vi "Habid_2-D_Histogram_Max_Average_and_Derivate_Beta.vi"() -> ()   [LabVIEW 2009]
uses:
  <vilib>/Analysis/6fits.llb/Curve Fitting Criteria.ctl
  <vilib>/Utility/file.llb/Write To Spreadsheet File (DBL).vi
  <vilib>/Analysis/3filter.llb/Savitzky-Golay Filter (DBL).vi
  <vilib>/Analysis/3filter.llb/Butterworth Filter (DBL).vi
  <vilib>/Analysis/NI_AALBase.lvlib
  <vilib>/Analysis/NI_AALPro.lvlib
  <vilib>/ptbypt/NI_PtbyPt.lvlib
panel:
  out "derivative M.A. 2":cluster{"Filtered X":dbl[], dbl[]}(graph)
  in  "Save 2-D":bool
  in  "Result File Dir 3":path
  in  "Result File Name 3":string="1D_Histogram.txt"
  out "y-axis":dbl[](array[numeric])
  out "S.D.":dbl format="%0.2f"
  in  "AC Mod Gain":dbl=5.0
  out "x-axis":dbl[](array[numeric])
  in  "Save 1-D":bool
  in  "Result File Dir":path
  in  "Result File Name":string="1D_Histogram.txt"
  in  "Save Derivative?":bool
  in  "Result File Dir 2":path
  in  "Result File Name 2":string="1D_Histogram.txt"
  in  "Ramp Rate":dbl=5.0
  out "Individual 2D Histogram":dbl[][](graph)
  out "Total 2D Histogram":dbl[][](graph)
  out "derivative M.A.":cluster{"Value":dbl, dbl, dbl[]}(graph)
  out "Smooth M.A.":cluster{"Value":dbl, dbl, dbl[]}(graph)
  in  "polynomial order 2":i32=3
  in  "side points 2":i32=9
  out "fit for M.A 2":cluster{"Value":dbl, dbl, dbl[][]}(graph)
  out "slope M.A.":dbl
  out "Real Threshold M.A.":cluster{"Value":dbl, dbl, dbl[]}(graph)
  in  "threshold y 2":dbl=-2.0
  out "Threshold 2":cluster{"Value":dbl, dbl, dbl[]}(graph)
  out "fit for M.A.":cluster{"Value":dbl, dbl, dbl[]}(graph)
  out "1-D Histogram M.A.":cluster{dbl[], dbl[]}[](graph)
  in  "Average Max?":bool
  in  "Threshold?":bool
  in  "Derivative?":bool
  out "fit for Max":cluster{"Value":dbl, dbl, dbl[]}(graph)
  out "S.D. Fit":dbl format="%0.5f"
  out "threshold slope":dbl
  out "fit threshold":cluster{dbl, dbl, ext[][]}(graph)
  out "threshold":cluster{dbl, dbl, ext[]}(graph)
  out "mean":dbl format="%0.5f"
  out "slope":dbl
  out "Fit":cluster{dbl, dbl, ext[][]}(graph)
  out "Gain Multiplier I(t)":cluster{dbl, dbl, "Filtered X":dbl[]}(graph)
  out "After I(t)":cluster{dbl, dbl, "Filtered X":dbl[]}(graph)
  out "Before I(t)":cluster{dbl, "SamplingTime":dbl, "Data":ext[]}(graph)
  in  "start path":path=path "J:/data"
  out "NormAC":dbl[](array[numeric])
  in  "Save Curve?":bool
  out "CurrentFileName":string
  out "SelectedCurves":i32
  out "CurvesInHistogram":bool[](array[boolean])
  out "1-D Histogram":cluster{dbl[], dbl[]}(graph)
  in  "1-D Histogram?":bool
  in  "Continuous?":bool
  in  "Add Histogram?":bool
  in  "Current (V) bins":i32=100
  in  "Current (V) max":dbl=2.0
  in  "Current (V) min":dbl=-3.0
  in  "Distance bins":i32=500
  in  "Distance max":dbl=4.0
  in  "Distance min":dbl
  in  "+/-":bool=TRUE
  out "DcData":dbl[](array[numeric])
  out "Beta":dbl[](array[numeric])
  out "DcDataLog":dbl[](array[numeric])
  out "TotalCurves":i32
  out "CurrentCurve":i32
  in  "Next Curve":bool
  in  "Previous Curve":bool
  out "AC I(t)":T1(graph)
  in  "Piezo Sensitivity (nm/V)":dbl=3.89
  in  "Z-mod Amp (V)":dbl=0.0257
  in  "Gac/Gdc":dbl=1.16618
  in  "low cutoff freq: fl":u32=600
  in  "high cutoff freq: fh":u32=1400
  out "DC I(t)":T2(graph)
  in  "DC cutoff freq":i32=1200
  out "Original I(t)":cluster{dbl, "SamplingTime":dbl, "Data":ext[]}(graph)
  out "DataBuffer":dbl[](array[numeric])
  out "Sampling Freq":dbl
  out "Sampling Time":dbl
  out "TimeLine":dbl[](array[numeric])
  in  "stop":bool
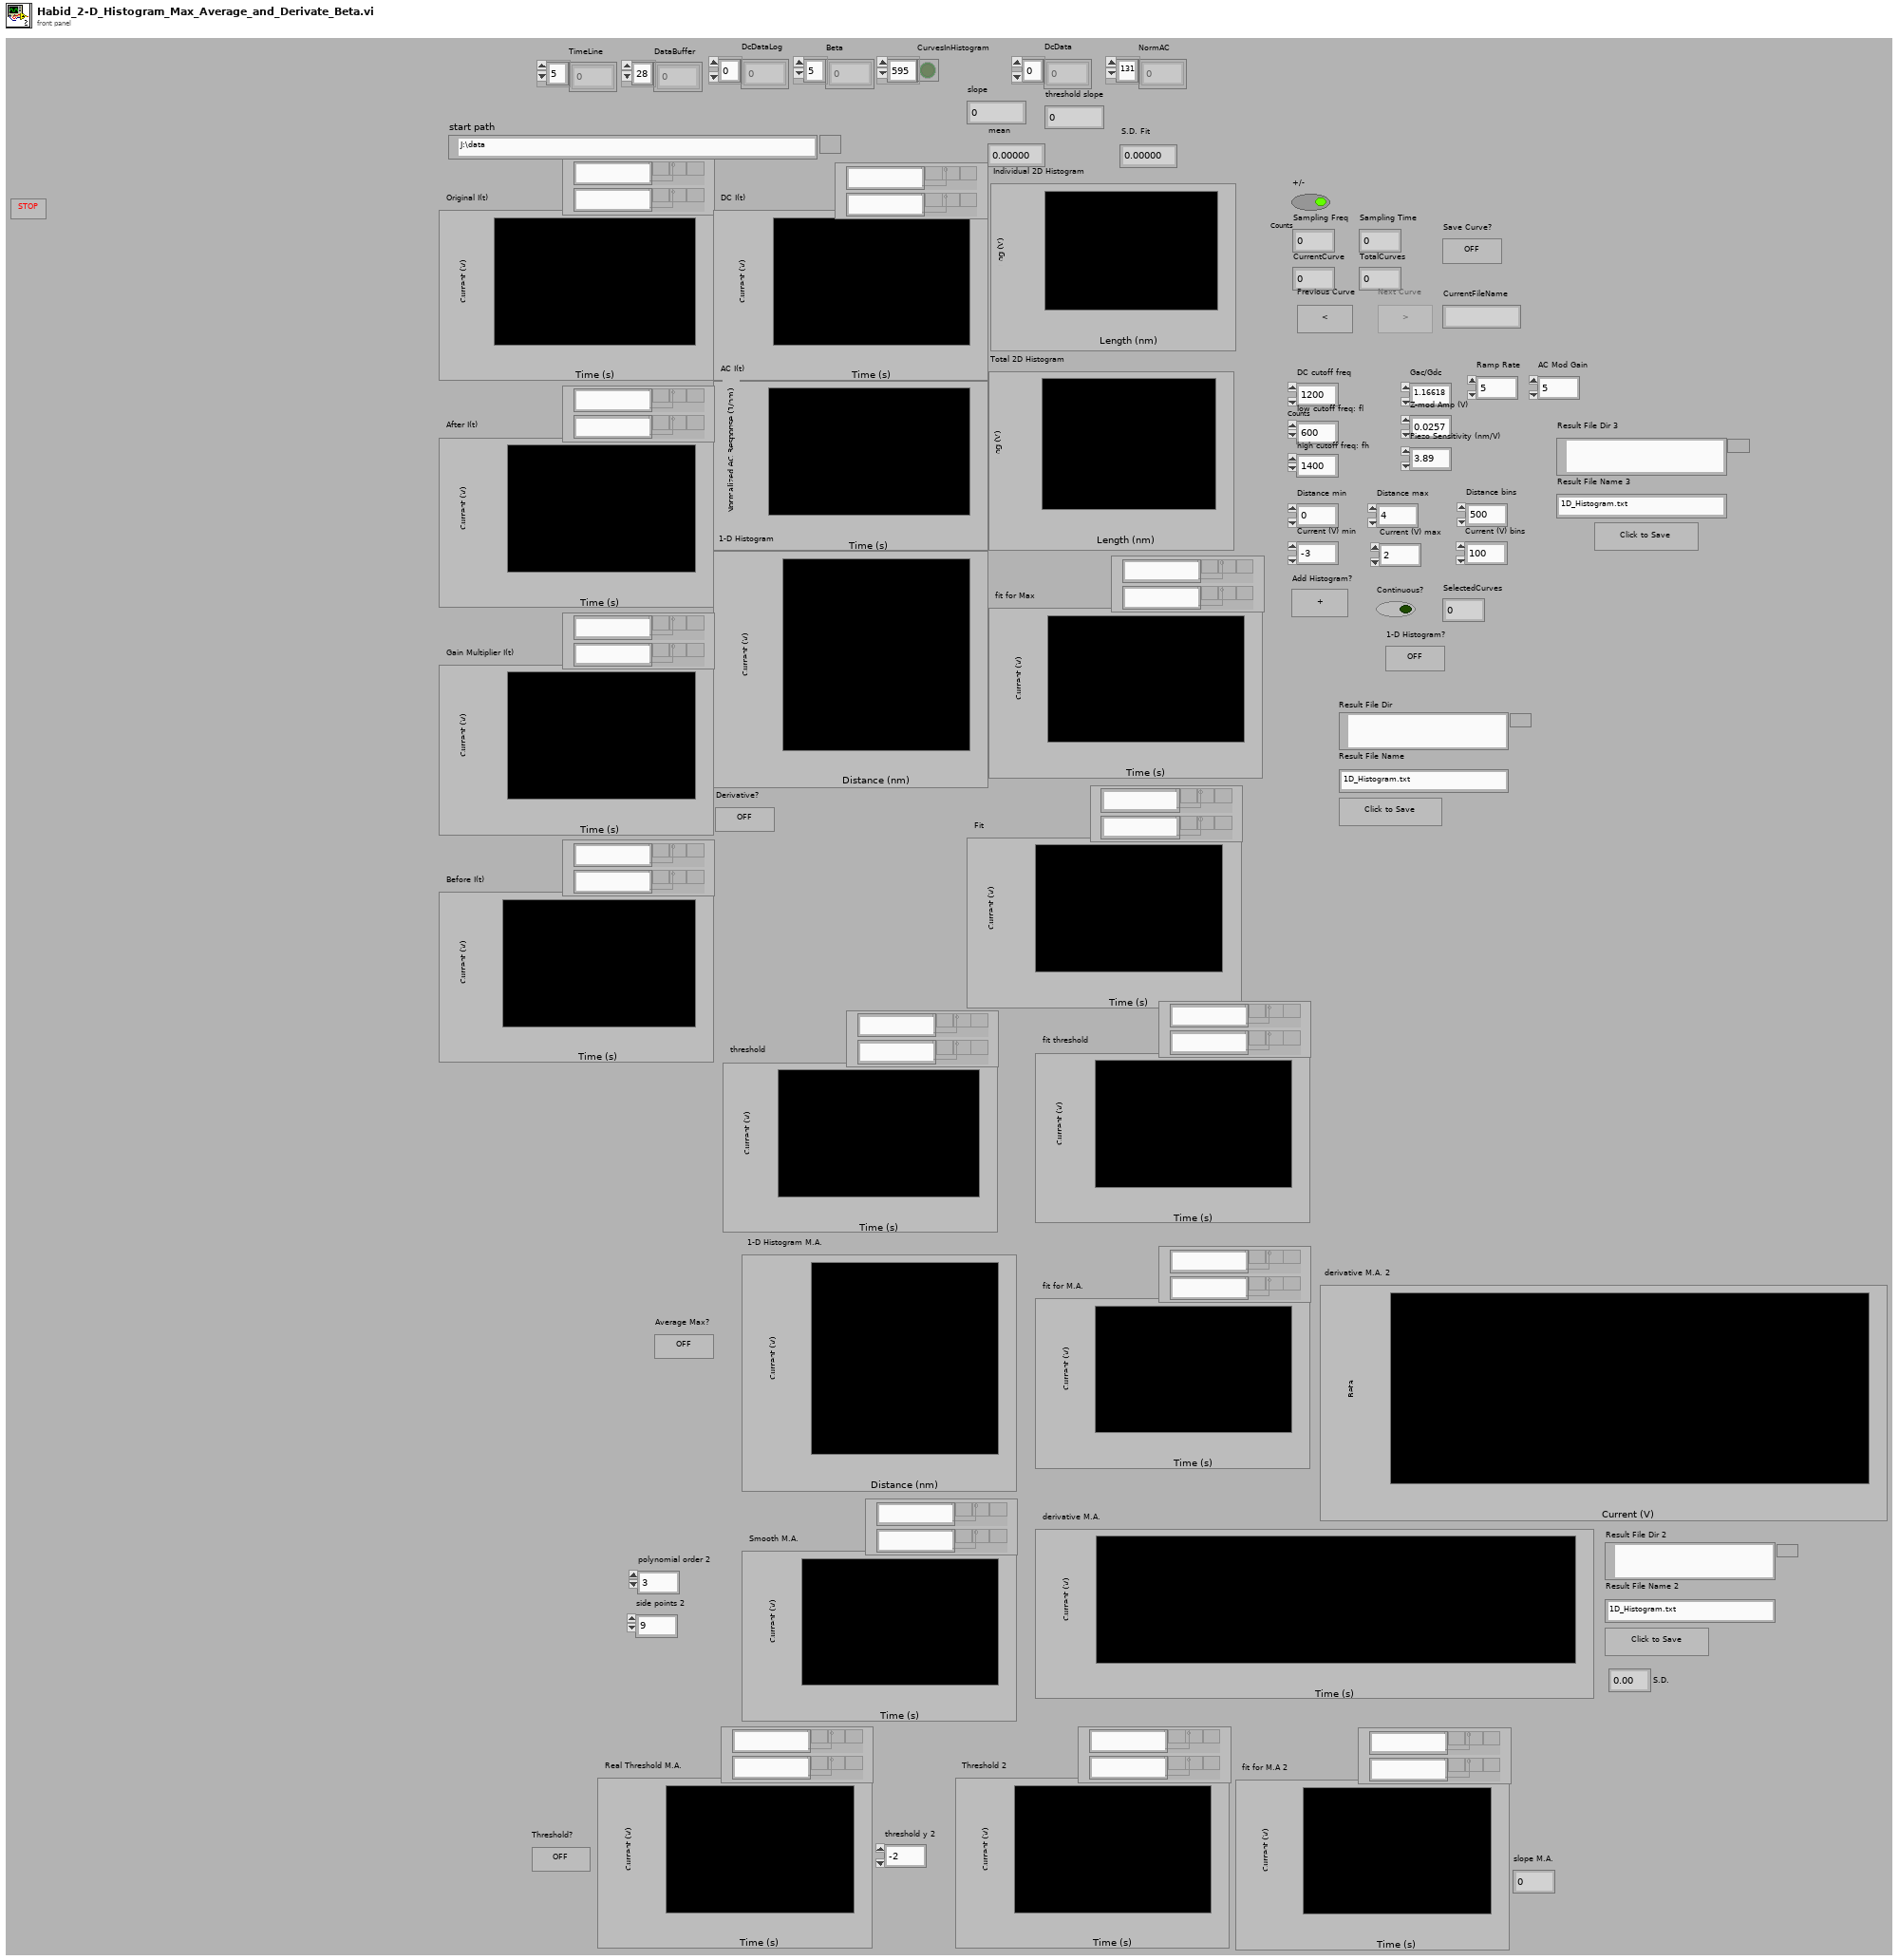
[diagram p1: front panel]
types:
  T1 = cluster{"Start Time":dbl, "Sampling Time":dbl, dbl[][]}
  T2 = cluster{dbl, "SamplingTime":dbl, "Filtered X":dbl[]}
  T3 = enum32{"Lowpass", "Highpass", "Bandpass", "Bandstop"}
  T4 = typedef "NI_AALPro.lvlib/Curve Fitting Criteria.ctl" = u16
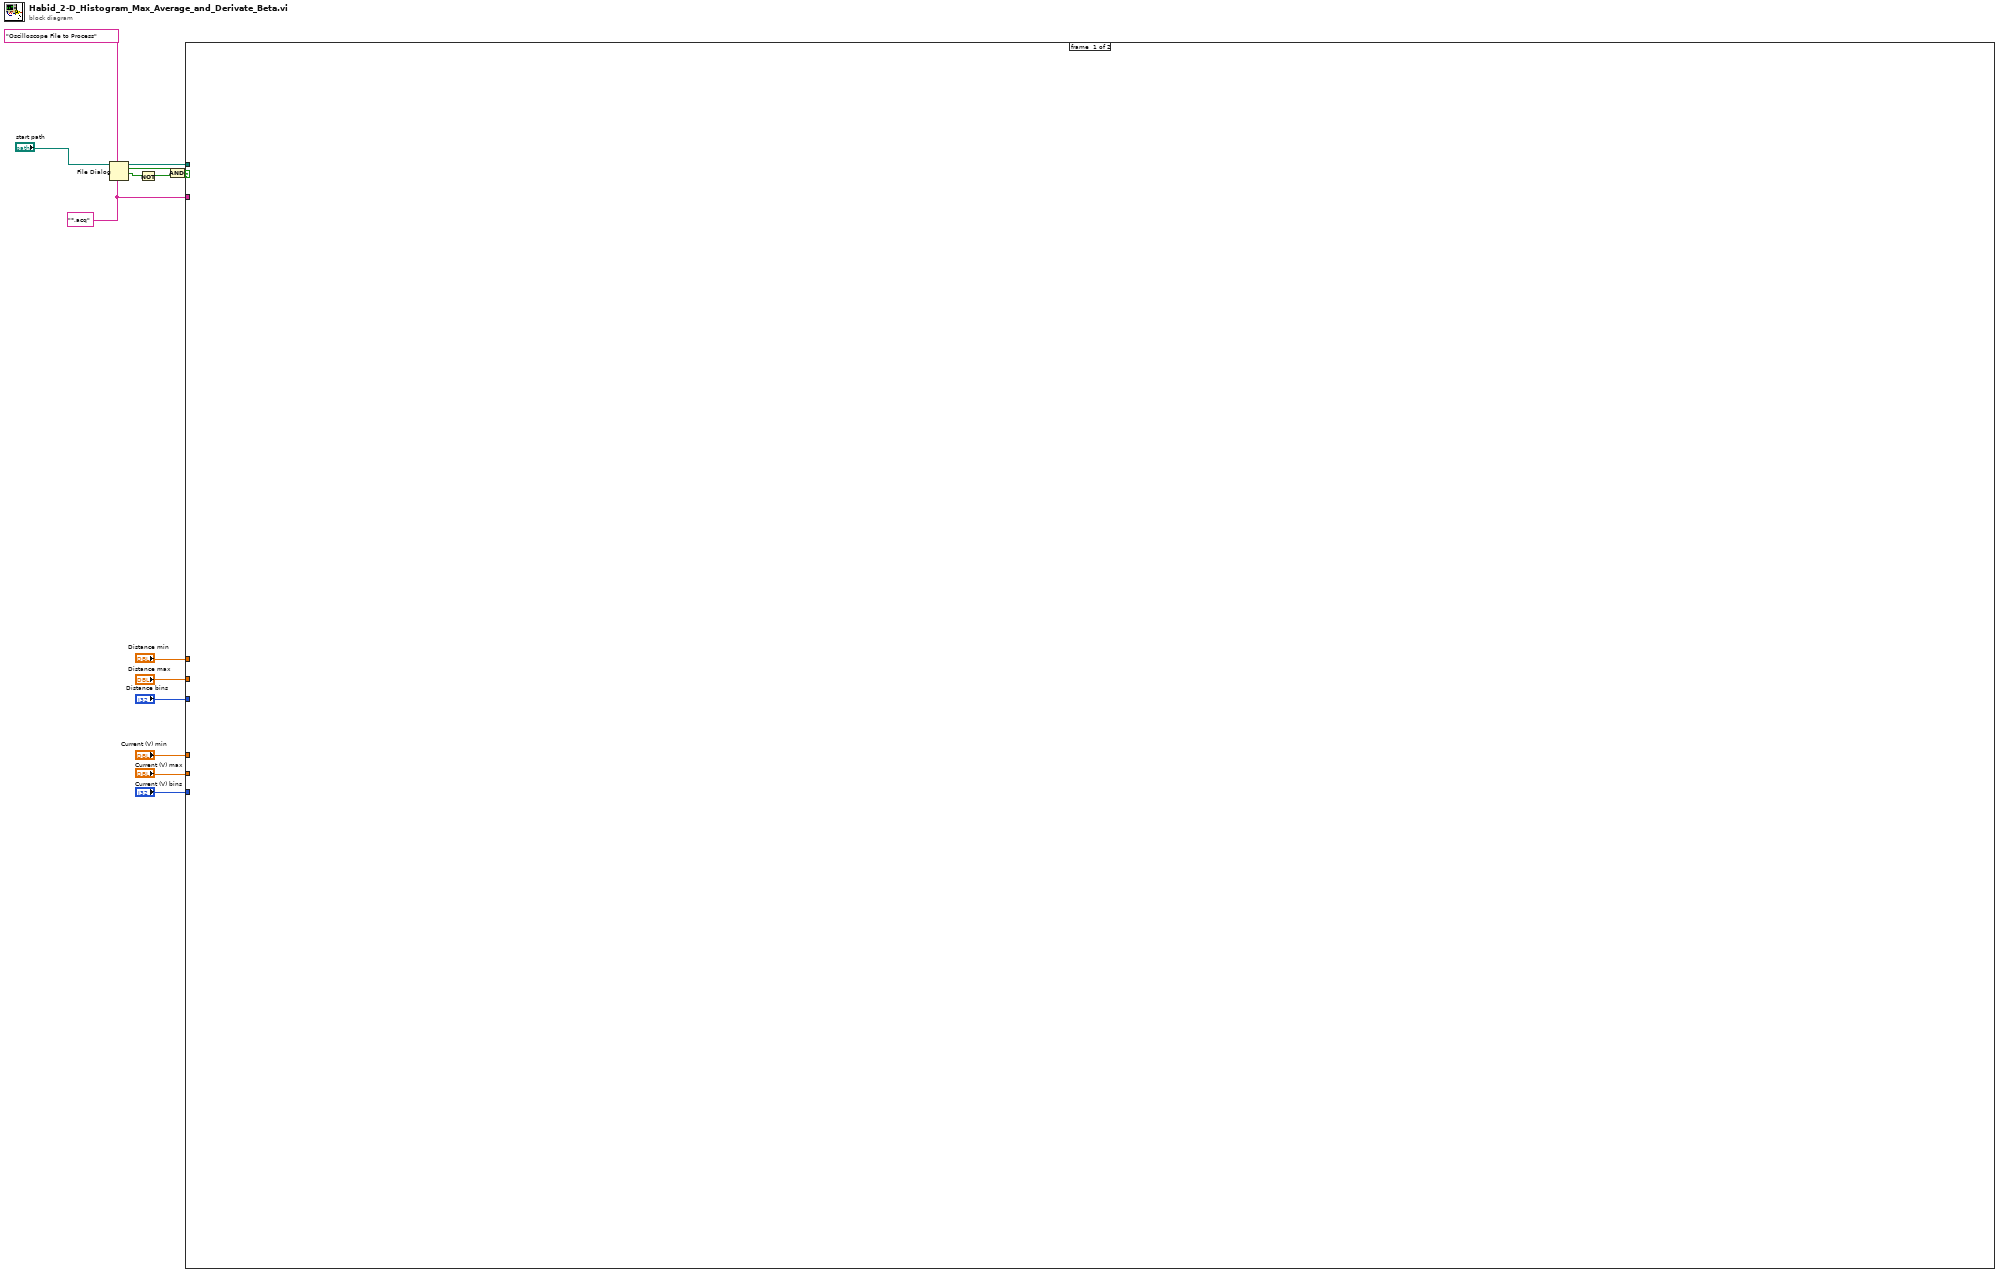
[diagram p0: block diagram]
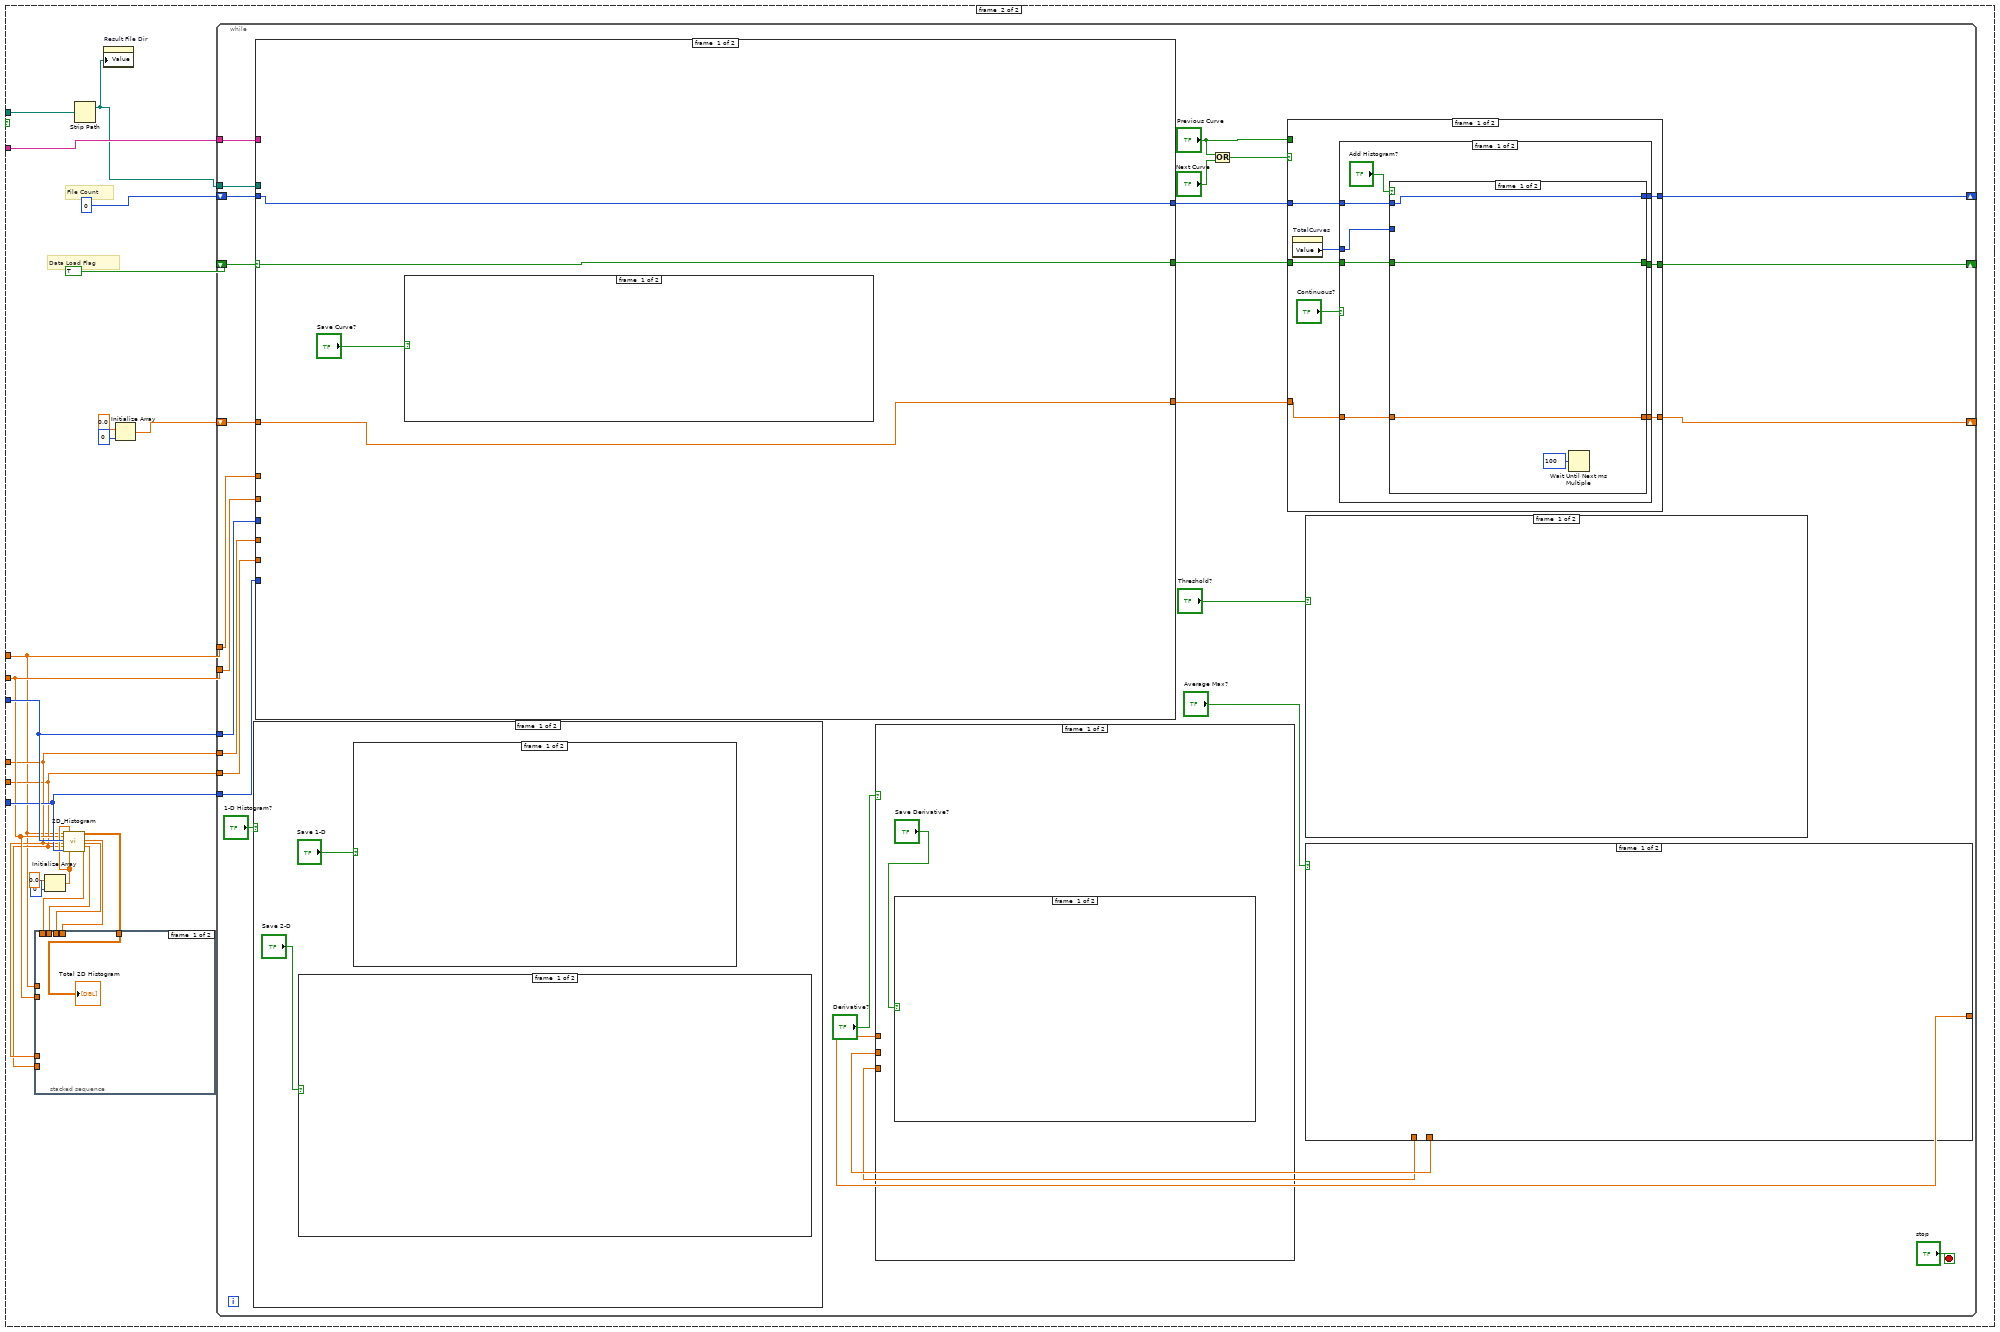
[diagram p2: hidden frame]
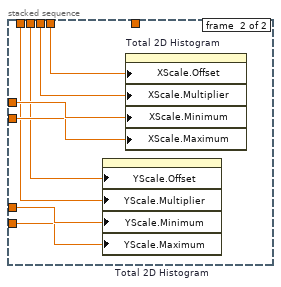
[diagram p3: hidden frame]
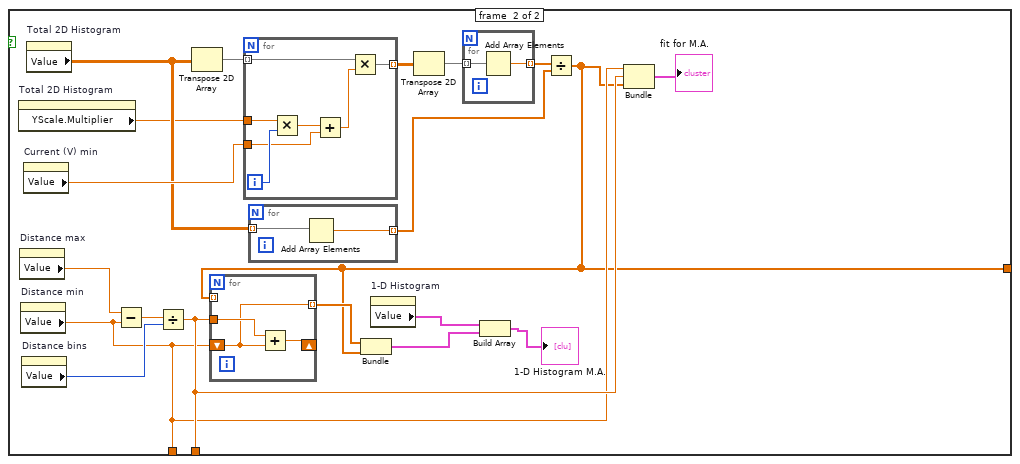
[diagram p4: hidden frame]
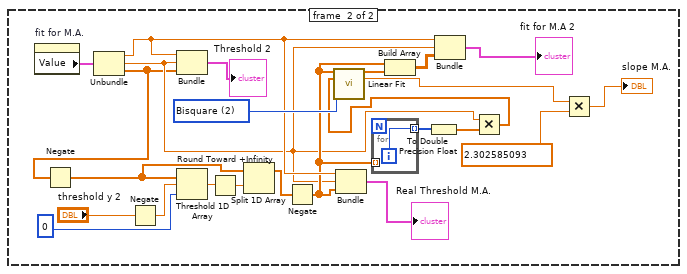
[diagram p5: hidden frame]
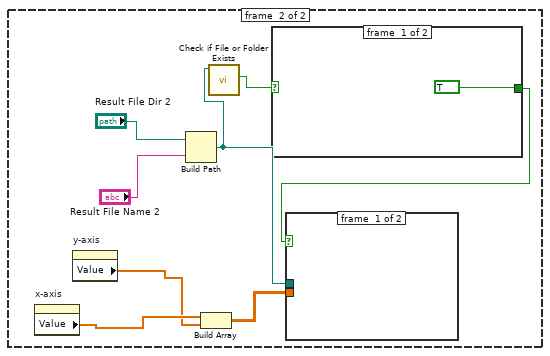
[diagram p6: hidden frame]
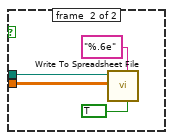
[diagram p7: hidden frame]
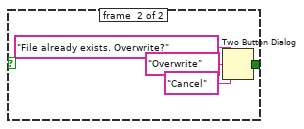
[diagram p8: hidden frame]
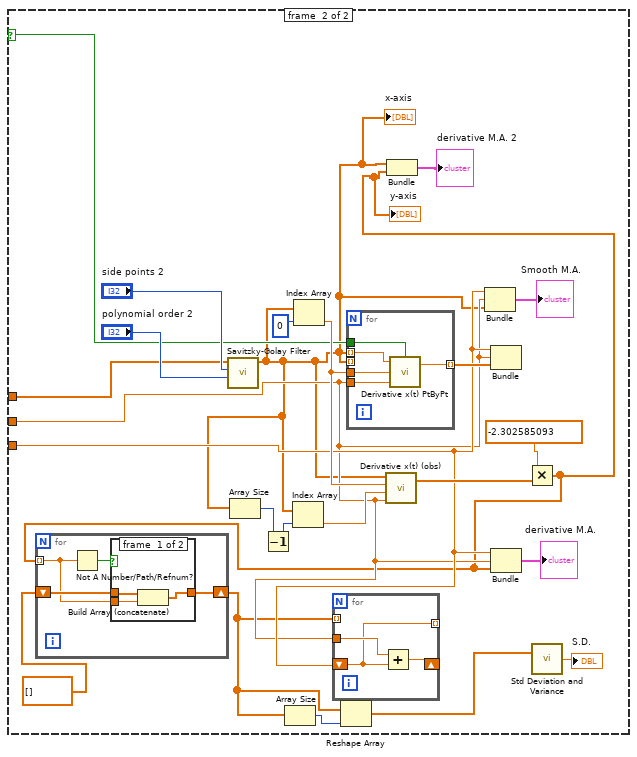
[diagram p9: hidden frame]
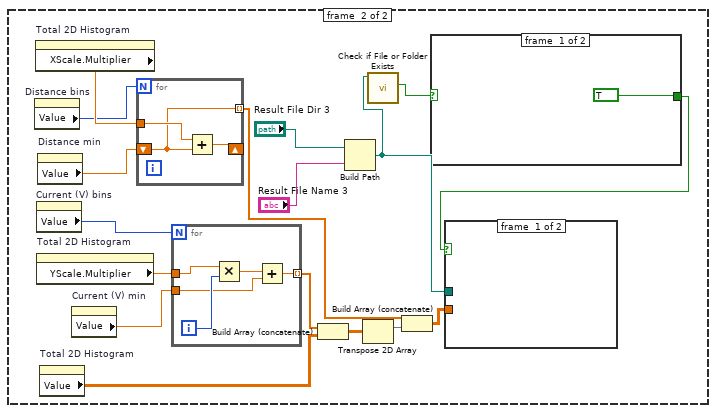
[diagram p11: hidden frame]
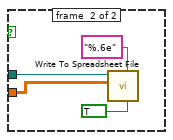
[diagram p12: hidden frame]
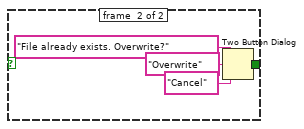
[diagram p13: hidden frame]
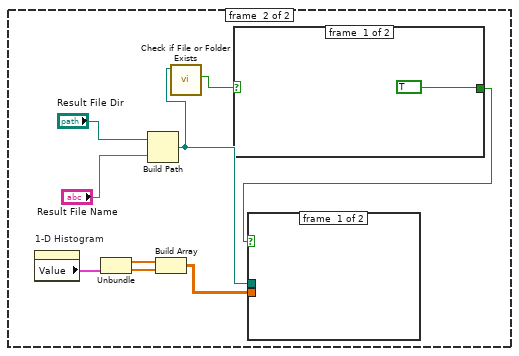
[diagram p14: hidden frame]
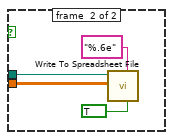
[diagram p15: hidden frame]
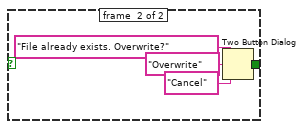
[diagram p16: hidden frame]
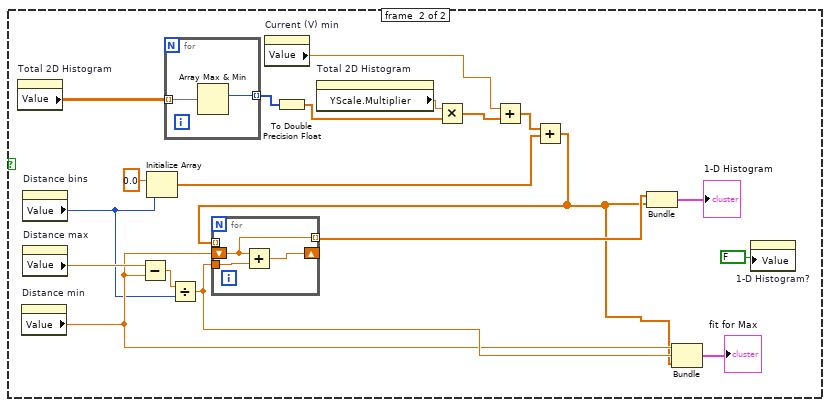
[diagram p17: hidden frame]
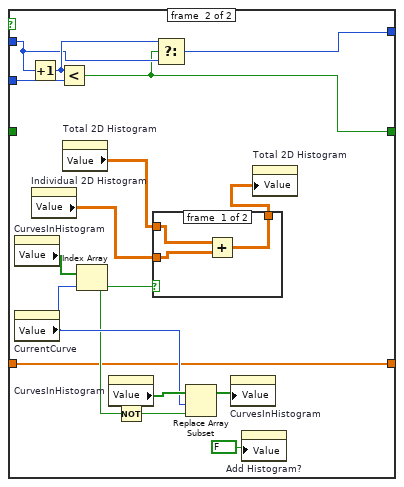
[diagram p18: hidden frame]
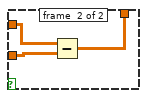
[diagram p19: hidden frame]
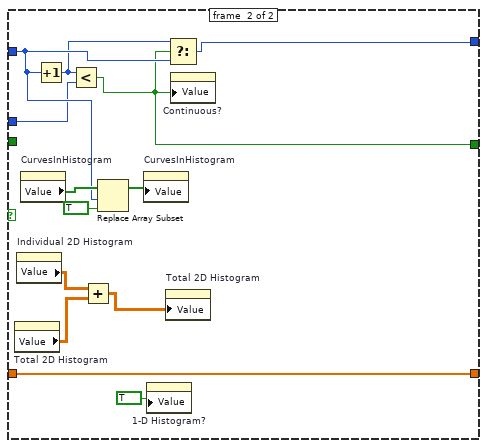
[diagram p20: hidden frame]
diagram:
  w7 = "*.acq" ("pattern (all files)")
  n1 = File Dialog(6:w7, 7:"Oscilloscope File to Process", 11:"start path") -> (1:w11:bool, 2:w13:bool, 3:w8:path)  [unwired: 4 in, 1 out]
  n2 = Not(x=w11) -> (.not. x?=w12:bool)
  n3 = And(x=w13, y=w12) -> (x .and. y?=w9:bool)
  n4 = case shown="True" w9 {
    tunnel: w8 -> [_ w36]
    tunnel: w7 -> [_ w34]
    tunnel: "Distance min" -> [_ w19]
    tunnel: "Distance max" -> [_ w22]
    tunnel: "Distance bins" -> [_ w32]
    tunnel: "Current (V) min" -> [_ w21]
    tunnel: "Current (V) max" -> [_ w20]
    tunnel: "Current (V) bins" -> [_ w31]
    frame #0 {
    }
    frame #1 {
      # "File Count"
      # "Data Load Flag"
      n5 = Initialize Array(0.0 ("element"), 0 ("dimension size")) -> (w23:dbl[])
      n6 = call "2D_Histogram.vi"("X min"=w19, "X max"=w22, "X bins"=w32, "Y min"=w21, "Y max"=w20, "Y bins"=w31, "X"=w23, "Y"=w23) -> ("X-Y 2-D Histogram"=w30:dbl[][], "Xoffset"=w29:dbl, "Xmultiplier"=w28:dbl, "Yoffset"=w27:dbl, "Ymultiplier"=w26:dbl)  [unwired: 7 in]
      n7 = stacked-sequence {
        tunnel: w30 -> [w37 _]
        tunnel: w28 -> [_ w44]
        tunnel: w26 -> [_ w40]
        tunnel: w29 -> [_ w45]
        tunnel: w27 -> [_ w41]
        tunnel: w19 -> [_ w43]
        tunnel: w22 -> [_ w42]
        tunnel: w21 -> [_ w39]
        tunnel: w20 -> [_ w38]
        frame #0 {
          "Total 2D Histogram" <- w37
        }
        frame #1 {
          n8 = property on="Total 2D Histogram" class="IntGraph (strict)"("YScale.Offset"=w41, "YScale.Multiplier"=w40, "YScale.Minimum"=w39, "YScale.Maximum"=w38) -> ()  [unwired: 2 in, 2 out]
          n9 = property on="Total 2D Histogram" class="IntGraph (strict)"("XScale.Offset"=w45, "XScale.Multiplier"=w44, "XScale.Minimum"=w43, "XScale.Maximum"=w42) -> ()  [unwired: 2 in, 2 out]
        }
      }
      n10 = Strip Path(path=w36) -> (stripped path=w15:path)  [unwired: 1 out]
      n11 = property on="Result File Dir" class="Path"("Value"=w15) -> ()  [unwired: 2 in, 2 out]
      n12 = Initialize Array(0.0 ("element"), 0 ("dimension size")) -> (w16:dbl[])
      n13 = while {
        shift-right: [w57] -> _
        shift-left: TRUE ("DataReload") -> [w72]
        tunnel: w34 -> [w71]
        tunnel: w15 -> [w47]
        shift-right: [w58] -> _
        shift-left: 0 -> [w70]
        tunnel: w19 -> [w67]
        tunnel: w22 -> [w66]
        tunnel: w32 -> [w65]
        tunnel: w21 -> [w64]
        tunnel: w20 -> [w63]
        tunnel: w31 -> [w62]
        shift-right: [w53] -> _
        shift-left: w16 -> [w55]
        stop <- "stop" stop-if-true
        n14 = case shown="False" "1-D Histogram?" {
          frame #0 {
            n15 = case shown="True" "Save 2-D" {
              frame #0 {
              }
              frame #1 {
                n16 = property on="Distance bins" class="DigNum (strict)"() -> ("Value"=w199:i32)  [unwired: 2 in, 2 out]
                n17 = property on="Total 2D Histogram" class="IntGraph (strict)"() -> ("XScale.Multiplier"=w200:dbl)  [unwired: 2 in, 2 out]
                n18 = property on="Current (V) bins" class="DigNum (strict)"() -> ("Value"=w203:i32)  [unwired: 2 in, 2 out]
                n19 = property on="Total 2D Histogram" class="IntGraph (strict)"() -> ("YScale.Multiplier"=w202:dbl)  [unwired: 2 in, 2 out]
                n20 = property on="Distance min" class="DigNum (strict)"() -> ("Value"=w198:dbl)  [unwired: 2 in, 2 out]
                n21 = property on="Total 2D Histogram" class="IntGraph (strict)"() -> ("Value"=w197:dbl[][])  [unwired: 2 in, 2 out]
                n22 = property on="Current (V) min" class="DigNum (strict)"() -> ("Value"=w201:dbl)  [unwired: 2 in, 2 out]
                n23 = for {
                  N: w199 -> [_]
                  tunnel: w200 -> [w211]
                  shift-right: [w210] -> _
                  shift-left: w198 -> [w209]
                  tunnel: [w209] -> w193 mode=indexing
                  n24 = Add(x=w211, y=w209) -> (x+y=w210:dbl)
                }
                n25 = for {
                  N: w203 -> [_]
                  tunnel: w202 -> [w214]
                  tunnel: w201 -> [w213]
                  tunnel: [w212] -> w196 mode=indexing
                  i -> [w215]
                  n26 = Multiply(x=w214, y=w215) -> (x*y=w216:dbl)
                  n27 = Add(x=w216, y=w213) -> (x+y=w212:dbl)
                }
                n28 = Build Array (concatenate)(w196, w197) -> (w195:dbl[][])
                n29 = Build Path(base path="Result File Dir 3", name or relative path="Result File Name 3") -> (appended path=w204:path)
                n30 = Transpose 2D Array(2D array=w195) -> (transposed array=w194:dbl[][])
                n31 = call <vilib>:"Check if File or Folder Exists.vi"("path"=w204) -> ("file or folder exists?"=w206:bool)  [unwired: 8 in, 2 out]
                n32 = Build Array (concatenate)(w193, w194) -> (w192:dbl[][])
                n33 = case shown="True" w206 {
                  tunnel: [TRUE ("T button?") w222] -> w205
                  frame #0 {
                  }
                  frame #1 {
                    n34 = Two Button Dialog(message="File already exists. Overwrite?", 1:"Cancel" ("F button name (\"Cancel\")"), 2:"Overwrite" ("T button name (\"OK\")")) -> (T button?=w222:bool)
                  }
                }
                n35 = case shown="True" w205 {
                  tunnel: w204 -> [_ w219]
                  tunnel: w192 -> [_ w217]
                  frame #0 {
                  }
                  frame #1 {
                    n36 = call-poly <vilib>:"Write To Spreadsheet File.vi"("transpose? (no:F)"=TRUE, "format (%.3f)"="%.6e", "2D data"=w217, "file path (dialog if empty)"=w219) -> ()  [unwired: 4 in, 1 out]
                  }
                }
              }
            }
            n37 = case shown="True" "Save 1-D" {
              frame #0 {
              }
              frame #1 {
                n38 = property on="1-D Histogram" class="XYGraph (strict)"() -> ("Value"=w234:cluster{dbl[], dbl[]})  [unwired: 2 in, 2 out]
                n39 = Unbundle(w234) -> (w233:dbl[], w232:dbl[])
                n40 = Build Path(base path="Result File Dir", name or relative path="Result File Name") -> (appended path=w227:path)
                n41 = Build Array(w233, w232) -> (w226:dbl[][])
                n42 = call <vilib>:"Check if File or Folder Exists.vi"("path"=w227) -> ("file or folder exists?"=w229:bool)  [unwired: 8 in, 2 out]
                n43 = case shown="True" w229 {
                  tunnel: [TRUE ("T button?") w240] -> w228
                  frame #0 {
                  }
                  frame #1 {
                    n44 = Two Button Dialog(message="File already exists. Overwrite?", 1:"Cancel" ("F button name (\"Cancel\")"), 2:"Overwrite" ("T button name (\"OK\")")) -> (T button?=w240:bool)
                  }
                }
                n45 = case shown="True" w228 {
                  tunnel: w226 -> [_ w236]
                  tunnel: w227 -> [_ w237]
                  frame #0 {
                  }
                  frame #1 {
                    n46 = call-poly <vilib>:"Write To Spreadsheet File.vi"("transpose? (no:F)"=TRUE, "format (%.3f)"="%.6e", "2D data"=w236, "file path (dialog if empty)"=w237) -> ()  [unwired: 4 in, 1 out]
                  }
                }
              }
            }
          }
          frame #1 {
            n47 = property on="Total 2D Histogram" class="IntGraph (strict)"() -> ("Value"=w246:dbl[][])  [unwired: 2 in, 2 out]
            n48 = property on="Distance min" class="DigNum (strict)"() -> ("Value"=w249:dbl)  [unwired: 2 in, 2 out]
            n49 = property on="Distance bins" class="DigNum (strict)"() -> ("Value"=w248:i32)  [unwired: 2 in, 2 out]
            n50 = property on="Distance max" class="DigNum (strict)"() -> ("Value"=w259:dbl)  [unwired: 2 in, 2 out]
            n51 = Subtract(x=w259, y=w249) -> (x-y=w261:dbl)
            n52 = Initialize Array(0.0 ("element"), w248) -> (w255:dbl[])
            n53 = for {
              tunnel: w246 -> [w264] mode=indexing
              tunnel: [w263] -> w257 mode=indexing
              n54 = Array Max & Min(array=w264) -> (max index (indices)=w263:i32)  [unwired: 3 out]
            }
            n55 = Divide(x=w261, y=w248) -> (x/y=w250:dbl)
            n56 = property on="Current (V) min" class="DigNum (strict)"() -> ("Value"=w251:dbl)  [unwired: 2 in, 2 out]
            n57 = To Double Precision Float(number=w257) -> (double precision float=w256:dbl[])
            n58 = property on="Total 2D Histogram" class="IntGraph (strict)"() -> ("YScale.Multiplier"=w245:dbl)  [unwired: 2 in, 2 out]
            n59 = Multiply(x=w245, y=w256) -> (x*y=w252:dbl[])
            n60 = Add(x=w251, y=w252) -> (x+y=w247:dbl[])
            n61 = Add(x=w247, y=w255) -> (x+y=w244:dbl[])
            n62 = for {
              shift-right: [w267] -> _
              shift-left: w249 -> [w265]
              tunnel: w250 -> [w266]
              tunnel: [w265] -> w254 mode=indexing
              tunnel: w244 -> [_] mode=indexing
              n63 = Add(x=w265, y=w266) -> (x+y=w267:dbl)
            }
            n64 = Bundle(w254, w244) -> (→"1-D Histogram":cluster{dbl[], dbl[]})  [unwired: 1 in]
            n65 = Bundle("Value"=w249, w250, w244) -> (→"fit for Max":cluster{"Value":dbl, dbl, dbl[]})  [unwired: 1 in]
            n66 = property on="1-D Histogram?" class="Bool (strict)"("Value"=FALSE ("1-D Histogram?")) -> ()  [unwired: 2 in, 2 out]
          }
        }
        n67 = case shown="True" w72 {
          selector: w72 -> [w336 _]
          tunnel: w71 -> [_ w473]
          tunnel: w70 -> [w335 w472]
          tunnel: [w336 FALSE] -> w69
          tunnel: [w335 w394] -> w68
          tunnel: w67 -> [_ w426]
          tunnel: w66 -> [_ w425]
          tunnel: w65 -> [_ w436]
          tunnel: w64 -> [_ w424]
          tunnel: w63 -> [_ w423]
          tunnel: w62 -> [_ w435]
          tunnel: w55 -> [w333 w392]
          tunnel: [w333 w367] -> w54
          tunnel: w47 -> [_ w355]
          frame #0 {
            n68 = case shown="True" "Save Curve?" {
              frame #0 {
              }
              frame #1 {
                n69 = property on="CurrentFileName" class="Str"() -> ("Value"=w348:string)  [unwired: 2 in, 2 out]
                n70 = property on="Result File Dir" class="Path"() -> ("Value"=w337:path)  [unwired: 2 in, 2 out]
                n71 = property on="TimeLine" class="Arr (strict)"() -> ("Value"=w342:dbl[])  [unwired: 2 in, 2 out]
                n72 = To Upper Case(1:w348) -> (0:w349:string)
                n73 = call <vilib>:"Search and Replace Pattern.vi"("string"=w349, "regular expression (\"\")"=".ACQ$" ("regular expression (\"\")"), "replace string (\"\")"=".txt" ("replace string (\"\")")) -> ("result string"=w347:string)  [unwired: 2 in, 1 out]
                n74 = property on="DataBuffer" class="Arr (strict)"() -> ("Value"=w341:dbl[])  [unwired: 2 in, 2 out]
                n75 = Build Path(base path=w337, name or relative path=w347) -> (appended path=w344:path)
                n76 = property on="DcData" class="Arr (strict)"() -> ("Value"=w340:dbl[])  [unwired: 2 in, 2 out]
                n77 = property on="NormAC" class="Arr (strict)"() -> ("Value"=w339:dbl[])  [unwired: 2 in, 2 out]
                n78 = property on="Beta" class="Arr (strict)"() -> ("Value"=w338:dbl[])  [unwired: 2 in, 2 out]
                n79 = Build Array(w342, w341, w340, w339, w338) -> (w343:dbl[][])
                n80 = call-poly <vilib>:"Write To Spreadsheet File.vi"("transpose? (no:F)"=TRUE, "format (%.3f)"="%.6e", "2D data"=w343, "file path (dialog if empty)"=w344) -> ()  [unwired: 4 in, 1 out]
              }
            }
          }
          frame #1 {
            w372 = T4 2 items=["Least Square", "Least Absolute Residual", "Bisquare"] ("method")
            w398 = T4 2 items=["Least Square", "Least Absolute Residual", "Bisquare"] ("method")
            w410 = 0.0
            n81 = First Call?() -> (First Call?: T/F=w434:bool)
            n82 = call "File_Browser.vi"("FileIndexIn"=w472, "FileExt"=w473, "FolderPath"=w355) -> ("Last?"=w449:bool, "FileIndexOut"=w394:i32, "FileTotal"=w433:i32, "FullFilePath"=w471:path, "First?"=w448:bool, "FileName"=→"CurrentFileName":string)  [unwired: 3 in]
            "CurrentCurve" <- w394
            "TotalCurves" <- w433
            n83 = Or(x=w448, y=w449) -> (x .or. y?=w452:bool)
            n84 = case shown="True" w434 {
              tunnel: w433 -> [_ w483]
              frame #0 {
              }
              frame #1 {
                n85 = Initialize Array(FALSE ("DataReload"), w483) -> (→"CurvesInHistogram":bool[])
              }
            }
            n86 = case shown="True" w452 {
              tunnel: w448 -> [_ w513]
              tunnel: [0 w512] -> w450
              tunnel: [0 w511] -> w451
              frame #0 {
              }
              frame #1 {
                # "Button Control:"
                n87 = case shown="True" w513 {
                  tunnel: [0 2] -> w512
                  tunnel: [2 0] -> w511
                  frame #0 {
                  }
                  frame #1 {
                  }
                }
              }
            }
            n88 = call "Acq_Reader.vi"("AcqFileToRead"=w471) -> ("SamplingFreq"=w447:dbl, "Data"=w445:ext[], "TimeLine"=→"TimeLine":dbl[])  [unwired: 8 in]
            "Sampling Freq" <- w447
            n89 = Reciprocal(x=w447) -> (1/x=w400:dbl)
            "Sampling Time" <- w400
            n90 = Negate(x=w445) -> (-x=w444:ext[])
            n91 = property on="Previous Curve" class="Bool"("Disabled"=w450) -> ()  [unwired: 2 in, 2 out]
            n92 = property on="Next Curve" class="Bool"("Disabled"=w451) -> ()  [unwired: 2 in, 2 out]
            n93 = Select(t=w445, s="+/-", f=w444) -> (s? t:f=w446:ext[])
            n94 = while {
              shift-right: [w498] -> w354
              shift-left: w446 -> [w499]
              stop <- w500 continue-if-true
              n95 = Array Max & Min(array=w499) -> (min value=w502:ext, min index (indices)=w501:i32)  [unwired: 2 out]
              n96 = Less Or Equal?(x=w502, y=0) -> (x <= y?=w500:bool)
              n97 = case shown="True" w500 {
                tunnel: w501 -> [_ w508]
                tunnel: w499 -> [w504 w507]
                tunnel: [w504 w506] -> w498
                frame #0 {
                }
                frame #1 {
                  n98 = Replace Array Subset(array=w507, new element=ext 0.00000100000000000000000004 ("new element/subarray"), index=w508) -> (w506:ext[])
                }
              }
            }
            "DataBuffer" <- w354
            n99 = Bundle(0.0, w400, "Data"=w354) -> (→"Before I(t)":cluster{dbl, dbl, "Data":ext[]})  [unwired: 1 in]
            n100 = Bundle(w410, w400, "Data"=w354) -> (→"Original I(t)":cluster{dbl, dbl, "Data":ext[]})  [unwired: 1 in]
            n101 = Multiply(x=w354, y="AC Mod Gain") -> (x*y=w353:ext[])
            n102 = call-poly <vilib>:"Butterworth Filter.vi"("init/cont (init:F)"=TRUE, "order"=4, "filter type"=T3."Lowpass", "low cutoff freq: fl"="DC cutoff freq", "sampling freq: fs"=w447, "X"=w354) -> ("Filtered X"=w357:dbl[])  [unwired: 2 in, 1 out]
            "DcData" <- w357
            n103 = call-poly <vilib>:"Butterworth Filter.vi"("init/cont (init:F)"=TRUE, "filter type"=T3."Bandpass", "low cutoff freq: fl"="low cutoff freq: fl", "high cutoff freq: fh"="high cutoff freq: fh", "sampling freq: fs"=w447, "X"=w353) -> ("Filtered X"=w412:dbl[])  [unwired: 2 in, 1 out]
            n104 = Compound Arithmetic op=MULTIPLY(w412, "Gac/Gdc") -> (w409:dbl[])
            n105 = Logarithm Base 10(1:w357) -> (0:→"DcDataLog":dbl[])
            n106 = property on="CurvesInHistogram" class="Arr (strict)"() -> ("Value"=w428:bool[])  [unwired: 2 in, 2 out]
            n107 = Compound Arithmetic op=MULTIPLY("Z-mod Amp (V)", "Piezo Sensitivity (nm/V)") -> (w459:dbl)
            n108 = flat-sequence {
              tunnel: w441 -> [w485]
              tunnel: w426 -> [w489]
              tunnel: w425 -> [w488]
              tunnel: w424 -> [w487]
              tunnel: w423 -> [w486]
              tunnel: [w489] -> w422
              tunnel: [w488] -> w421
              tunnel: [w487] -> w420
              tunnel: [w486] -> w419
              tunnel: w440 -> [w496]
              tunnel: w439 -> [w492]
              tunnel: w438 -> [w497]
              tunnel: w437 -> [w493]
              tunnel: w422 -> [w495]
              tunnel: w421 -> [w494]
              tunnel: w420 -> [w491]
              tunnel: w419 -> [w490]
              frame #0 {
                "Individual 2D Histogram" <- w485
              }
              frame #1 {
                n109 = property on="Individual 2D Histogram" class="IntGraph (strict)"("XScale.Offset"=w497, "XScale.Multiplier"=w496, "XScale.Minimum"=w495, "XScale.Maximum"=w494) -> ()  [unwired: 2 in, 2 out]
                n110 = property on="Individual 2D Histogram" class="IntGraph (strict)"("YScale.Offset"=w493, "YScale.Multiplier"=w492, "YScale.Minimum"=w491, "YScale.Maximum"=w490) -> ()  [unwired: 2 in, 2 out]
              }
            }
            n111 = Bundle(w410, w400, "Filtered X"=w357) -> (→"DC I(t)":cluster{dbl, dbl, "Filtered X":dbl[]})  [unwired: 1 in]
            n112 = Divide(x=w409, y=w459) -> (x/y=w454:dbl[])
            "NormAC" <- w454
            n113 = Multiply(x="Ramp Rate", y=3.89) -> (x*y=w401:dbl)
            n114 = Index Array(array=w428, index=w394) -> (element=w432:bool)
            n115 = call <vilib>:"Fast Hilbert Transform.vi"("X"=w454) -> ("Hilbert{X}"=w458:dbl[])  [unwired: 1 out]
            n116 = Re/Im To Complex(1:w458, 2:w454) -> (0:w457:cdb[])
            n117 = case shown="False" w432 {
              tunnel: [string[] ["+", "+", "+", "+"] ("Strings [4]") string[] ["-", "-", "-", "-"] ("Strings [4]")] -> w431
              frame #0 {
              }
              frame #1 {
              }
            }
            n118 = Multiply(x=w401, y=w400) -> (x*y=w360:dbl)
            n119 = Absolute Value(x=w457) -> (abs(x)=w442:dbl[])
            "Beta" <- w442
            n120 = Build Array(w442, w454) -> (w456:dbl[][])
            n121 = Bundle(w410, w400, w409) -> (→"Gain Multiplier I(t)":cluster{dbl, dbl, dbl[]})  [unwired: 1 in]
            n122 = Bundle(w410, w400, w456) -> (→"AC I(t)":cluster{dbl, dbl, dbl[][]})  [unwired: 1 in]
            n123 = Array Size(array=w428) -> (size(s)=w430:i32)
            n124 = Bundle(w410, w400, "Filtered X"=w412) -> (→"After I(t)":cluster{dbl, dbl, "Filtered X":dbl[]})  [unwired: 1 in]
            n125 = for {
              N: w430 -> [_]
              shift-right: [w476] -> w427
              shift-left: 0 -> [w478]
              tunnel: w428 -> [w479] mode=indexing
              n126 = Increment(x=w478) -> (x+1=w477:i32)
              n127 = Select(t=w477, s=w479, f=w478) -> (s? t:f=w476:i32)
            }
            "SelectedCurves" <- w427
            n128 = property on="Add Histogram?" class="Bool (strict)"("Strings [4]"=w431) -> ()  [unwired: 2 in, 2 out]
            n129 = for {
              tunnel: [w475] -> w408 mode=indexing
              tunnel: w354 -> [_] mode=indexing
              i -> [w475]
            }
            n130 = Multiply(x=w354, y=1e-08) -> (x*y=w396:ext[])
            n131 = To Double Precision Float(number=w408) -> (double precision float=w407:dbl[])
            n132 = Natural Logarithm(1:w396) -> (0:w356:ext[])
            n133 = Multiply(x=w407, y=w360) -> (x*y=w368:dbl[])
            n134 = call <vilib>:"Linear Fit.vi"("Y"=w356, "X"=w368, "method"=w398) -> ("Best Linear Fit"=w397:dbl[], "slope"=w395:dbl)  [unwired: 8 in, 3 out]
            "slope" <- w395
            n135 = Build Array(w356, w397) -> (w404:ext[][])
            n136 = Insert Into Array(array=w392, index=w394, new element=w395) -> (w367:dbl[])
            n137 = Bundle(0.0, w360, w404) -> (→"Fit":cluster{dbl, dbl, ext[][]})  [unwired: 1 in]
            n138 = call <vilib>:"Mean.vi"("X"=w367) -> ("mean"=→"mean":dbl)  [unwired: 1 out]
            n139 = Reverse 1D Array(array=w354) -> (reversed array=w359:ext[])
            n140 = Threshold 1D Array(1:0 ("start index (0)"), 2:ext 10.0 ("threshold y"), 3:w359) -> (0:w386:ext)
            n141 = Round Toward +Infinity(x=w386) -> (ceil(x): smallest int >= x=w387:ext)
            n142 = Reverse 1D Array(array=w354) -> (reversed array=w388:ext[])
            n143 = call <vilib>:"Std Deviation and Variance.vi"("X"=w367) -> ("standard deviation"=→"S.D. Fit":dbl)  [unwired: 1 in, 2 out]
            n144 = Split 1D Array(array=w388, index=w387) -> (first subarray=w384:ext[])  [unwired: 1 out]
            n145 = Threshold 1D Array(1:0 ("start index (0)"), 2:0.005 ("threshold y"), 3:w384) -> (0:w377:ext)
            n146 = Round Toward -Infinity(1:w377) -> (0:w376:ext)
            n147 = Split 1D Array(array=w384, index=w376) -> (second subarray=w383:ext[])  [unwired: 1 out]
            n148 = Reverse 1D Array(array=w383) -> (reversed array=w365:ext[])
            n149 = Logarithm Base 10(1:w365) -> (0:w363:ext[])
            n150 = Multiply(x=1e-08, y=w365) -> (x*y=w379:ext[])
            n151 = for {
              tunnel: [w474] -> w375 mode=indexing
              tunnel: w365 -> [_] mode=indexing
              i -> [w474]
            }
            n152 = Natural Logarithm(1:w379) -> (0:w373:ext[])
            n153 = To Double Precision Float(number=w375) -> (double precision float=w374:dbl[])
            n154 = Multiply(x=w360, y=w374) -> (x*y=w362:dbl[])
            n155 = call "2D_Histogram.vi"("X min"=w426, "X max"=w425, "X bins"=w436, "Y min"=w424, "Y max"=w423, "Y bins"=w435, "X"=w362, "Y"=w363) -> ("X-Y 2-D Histogram"=w441:dbl[][], "Xoffset"=w438:dbl, "Xmultiplier"=w440:dbl, "Yoffset"=w437:dbl, "Ymultiplier"=w439:dbl)  [unwired: 7 in]
            n156 = call <vilib>:"Linear Fit.vi"("Y"=w373, "X"=w362, "method"=w372) -> ("Best Linear Fit"=w371:dbl[], "slope"=→"threshold slope":dbl)  [unwired: 8 in, 3 out]
            n157 = Bundle(0.0, w360, w365) -> (→"threshold":cluster{dbl, dbl, ext[]})  [unwired: 1 in]
            n158 = Build Array(w373, w371) -> (w370:ext[][])
            n159 = Bundle(0.0, w360, w370) -> (→"fit threshold":cluster{dbl, dbl, ext[][]})  [unwired: 1 in]
          }
        }
        n160 = Or(x="Previous Curve", y="Next Curve") -> (x .or. y?=w60:bool)
        n161 = case shown="False" w60 {
          selector: w60 -> [_ w325]
          tunnel: "Previous Curve" -> [_ w328]
          tunnel: w68 -> [w272 w327]
          tunnel: [w271 w326] -> w58
          tunnel: w69 -> [w275 _]
          tunnel: [w274 w325] -> w57
          tunnel: w54 -> [w269 w323]
          tunnel: [w268 w323] -> w53
          frame #0 {
            n162 = property on="TotalCurves" class="DigNum (strict)"() -> ("Value"=w270:i32)  [unwired: 2 in, 2 out]
            n163 = case shown="True" "Continuous?" {
              tunnel: w275 -> [w280 _]
              tunnel: [w279 w314] -> w274
              tunnel: w272 -> [w282 w319]
              tunnel: [w281 w322] -> w271
              tunnel: w270 -> [w278 w316]
              tunnel: w269 -> [w277 w313]
              tunnel: [w276 w313] -> w268
              frame #0 {
                n164 = case shown="True" "Add Histogram?" {
                  tunnel: w282 -> [w287 w294]
                  tunnel: [w287 w293] -> w281
                  tunnel: w280 -> [w286 _]
                  tunnel: [w286 w292] -> w279
                  tunnel: w278 -> [_ w296]
                  tunnel: w277 -> [w284 w291]
                  tunnel: [w284 w291] -> w276
                  frame #0 {
                    n165 = Wait Until Next ms Multiple(millisecond multiple=u32 100) -> ()  [unwired: 1 out]
                  }
                  frame #1 {
                    n166 = property on="CurvesInHistogram" class="Arr (strict)"() -> ("Value"=w302:bool[])  [unwired: 2 in, 2 out]
                    n167 = property on="CurrentCurve" class="DigNum (strict)"() -> ("Value"=w299:i32)  [unwired: 2 in, 2 out]
                    n168 = Increment(x=w294) -> (x+1=w295:i32)
                    n169 = property on="Individual 2D Histogram" class="IntGraph (strict)"() -> ("Value"=w288:dbl[][])  [unwired: 2 in, 2 out]
                    n170 = Less?(x=w295, y=w296) -> (x < y?=w292:bool)
                    n171 = property on="Total 2D Histogram" class="IntGraph (strict)"() -> ("Value"=w290:dbl[][])  [unwired: 2 in, 2 out]
                    n172 = Index Array(array=w302, index=w299) -> (element=w298:bool)
                    n173 = property on="CurvesInHistogram" class="Arr (strict)"() -> ("Value"=w301:bool[])  [unwired: 2 in, 2 out]
                    n174 = Not(x=w298) -> (.not. x?=w297:bool)
                    n175 = case shown="True" w298 {
                      tunnel: w290 -> [w306 w309]
                      tunnel: w288 -> [w305 w308]
                      tunnel: [w304 w307] -> w289
                      frame #0 {
                        n176 = Add(x=w306, y=w305) -> (x+y=w304:dbl[][])
                      }
                      frame #1 {
                        n177 = Subtract(x=w309, y=w308) -> (x-y=w307:dbl[][])
                      }
                    }
                    n178 = Select(t=w295, s=w292, f=w294) -> (s? t:f=w293:i32)
                    n179 = Replace Array Subset(array=w301, new element=w297, index=w299) -> (w300:bool[])
                    n180 = property on="CurvesInHistogram" class="Arr (strict)"("Value"=w300) -> ()  [unwired: 2 in, 2 out]
                    n181 = property on="Add Histogram?" class="Bool (strict)"("Value"=FALSE ("Add Histogram?")) -> ()  [unwired: 2 in, 2 out]
                    n182 = property on="Total 2D Histogram" class="IntGraph (strict)"("Value"=w289) -> ()  [unwired: 2 in, 2 out]
                  }
                }
              }
              frame #1 {
                n183 = property on="Total 2D Histogram" class="IntGraph (strict)"() -> ("Value"=w311:dbl[][])  [unwired: 2 in, 2 out]
                n184 = property on="Individual 2D Histogram" class="IntGraph (strict)"() -> ("Value"=w312:dbl[][])  [unwired: 2 in, 2 out]
                n185 = property on="CurvesInHistogram" class="Arr (strict)"() -> ("Value"=w320:bool[])  [unwired: 2 in, 2 out]
                n186 = Increment(x=w319) -> (x+1=w315:i32)
                n187 = Less?(x=w315, y=w316) -> (x < y?=w314:bool)
                n188 = Add(x=w312, y=w311) -> (x+y=w310:dbl[][])
                n189 = Replace Array Subset(array=w320, new element=TRUE ("new element/subarray"), index=w319) -> (w317:bool[])
                n190 = property on="CurvesInHistogram" class="Arr (strict)"("Value"=w317) -> ()  [unwired: 2 in, 2 out]
                n191 = property on="1-D Histogram?" class="Bool (strict)"("Value"=TRUE ("1-D Histogram?")) -> ()  [unwired: 2 in, 2 out]
                n192 = property on="Total 2D Histogram" class="IntGraph (strict)"("Value"=w310) -> ()  [unwired: 2 in, 2 out]
                n193 = Select(t=w315, s=w314, f=w319) -> (s? t:f=w322:i32)
                n194 = property on="Continuous?" class="Bool (strict)"("Value"=w314) -> ()  [unwired: 2 in, 2 out]
              }
            }
          }
          frame #1 {
            # "Curve Browse:"
            n195 = case shown="False" w328 {
              tunnel: w327 -> [w330 w332]
              tunnel: [w329 w331] -> w326
              frame #0 {
                n196 = Increment(x=w330) -> (x+1=w329:i32)
              }
              frame #1 {
                n197 = Decrement(x=w332) -> (x-1=w331:i32)
              }
            }
            n198 = property on="Continuous?" class="Bool (strict)"("Value"=FALSE ("Continuous?")) -> ()  [unwired: 2 in, 2 out]
          }
        }
        n199 = case shown="True" "Average Max?" {
          tunnel: [_ w74] -> w46
          tunnel: [_ w80] -> w49
          tunnel: [_ w79] -> w48
          frame #0 {
          }
          frame #1 {
            n200 = property on="Total 2D Histogram" class="IntGraph (strict)"() -> ("YScale.Multiplier"=w77:dbl)  [unwired: 2 in, 2 out]
            n201 = property on="Distance max" class="DigNum (strict)"() -> ("Value"=w91:dbl)  [unwired: 2 in, 2 out]
            n202 = property on="Distance min" class="DigNum (strict)"() -> ("Value"=w79:dbl)  [unwired: 2 in, 2 out]
            n203 = property on="Distance bins" class="DigNum (strict)"() -> ("Value"=w89:i32)  [unwired: 2 in, 2 out]
            n204 = property on="Current (V) min" class="DigNum (strict)"() -> ("Value"=w88:dbl)  [unwired: 2 in, 2 out]
            n205 = property on="Total 2D Histogram" class="IntGraph (strict)"() -> ("Value"=w78:dbl[][])  [unwired: 2 in, 2 out]
            n206 = Subtract(x=w91, y=w79) -> (x-y=w90:dbl)
            n207 = Divide(x=w90, y=w89) -> (x/y=w80:dbl)
            n208 = Transpose 2D Array(2D array=w78) -> (transposed array=w92:dbl[][])
            n209 = for {
              tunnel: w92 -> [w101] mode=indexing
              tunnel: w77 -> [w105]
              tunnel: w88 -> [w103]
              tunnel: [w100] -> w87 mode=indexing
              i -> [w106]
              n210 = Multiply(x=w105, y=w106) -> (x*y=w104:dbl)
              n211 = Add(x=w104, y=w103) -> (x+y=w102:dbl)
              n212 = Multiply(x=w101, y=w102) -> (x*y=w100:dbl[])
            }
            n213 = for {
              tunnel: w78 -> [w97] mode=indexing
              tunnel: [w96] -> w85 mode=indexing
              n214 = Add Array Elements(numeric array=w97) -> (sum=w96:dbl)
            }
            n215 = property on="1-D Histogram" class="XYGraph (strict)"() -> ("Value"=w82:cluster{dbl[], dbl[]})  [unwired: 2 in, 2 out]
            n216 = Transpose 2D Array(2D array=w87) -> (transposed array=w86:dbl[][])
            n217 = for {
              tunnel: w86 -> [w99] mode=indexing
              tunnel: [w98] -> w84 mode=indexing
              n218 = Add Array Elements(numeric array=w99) -> (sum=w98:dbl)
            }
            n219 = Divide(x=w84, y=w85) -> (x/y=w74:dbl[])
            n220 = for {
              tunnel: w74 -> [_] mode=indexing
              tunnel: w80 -> [w95]
              shift-right: [w94] -> _
              shift-left: w79 -> [w93]
              tunnel: [w93] -> w75 mode=indexing
              n221 = Add(x=w95, y=w93) -> (x+y=w94:dbl)
            }
            n222 = Bundle(w75, w74) -> (w76:cluster{dbl[], dbl[]})  [unwired: 1 in]
            n223 = Build Array(w82, w76) -> (→"1-D Histogram M.A.":cluster{dbl[], dbl[]}[])
            n224 = Bundle("Value"=w79, w80, w74) -> (→"fit for M.A.":cluster{"Value":dbl, dbl, dbl[]})  [unwired: 1 in]
          }
        }
        n225 = case shown="True" "Derivative?" {
          selector: "Derivative?" -> [_ w163]
          tunnel: w46 -> [_ w162]
          tunnel: w49 -> [_ w158]
          tunnel: w48 -> [_ w159]
          frame #0 {
            n226 = case shown="True" "Save Derivative?" {
              frame #0 {
              }
              frame #1 {
                n227 = property on="x-axis" class="Arr (strict)"() -> ("Value"=w134:dbl[])  [unwired: 2 in, 2 out]
                n228 = property on="y-axis" class="Arr (strict)"() -> ("Value"=w133:dbl[])  [unwired: 2 in, 2 out]
                n229 = Build Path(base path="Result File Dir 2", name or relative path="Result File Name 2") -> (appended path=w136:path)
                n230 = Build Array(w134, w133) -> (w135:dbl[][])
                n231 = call <vilib>:"Check if File or Folder Exists.vi"("path"=w136) -> ("file or folder exists?"=w138:bool)  [unwired: 8 in, 2 out]
                n232 = case shown="True" w138 {
                  tunnel: [TRUE ("T button?") w146] -> w137
                  frame #0 {
                  }
                  frame #1 {
                    n233 = Two Button Dialog(message="File already exists. Overwrite?", 1:"Cancel" ("F button name (\"Cancel\")"), 2:"Overwrite" ("T button name (\"OK\")")) -> (T button?=w146:bool)
                  }
                }
                n234 = case shown="True" w137 {
                  tunnel: w135 -> [_ w142]
                  tunnel: w136 -> [_ w143]
                  frame #0 {
                  }
                  frame #1 {
                    n235 = call-poly <vilib>:"Write To Spreadsheet File.vi"("transpose? (no:F)"=TRUE, "format (%.3f)"="%.6e", "2D data"=w142, "file path (dialog if empty)"=w143) -> ()  [unwired: 4 in, 1 out]
                  }
                }
              }
            }
          }
          frame #1 {
            n236 = call-poly <vilib>:"Savitzky-Golay Filter.vi"("polynomial order"="polynomial order 2", "side points"="side points 2", "X"=w162) -> ("Filtered X"=w150:dbl[])  [unwired: 7 in, 1 out]
            "x-axis" <- w150
            n237 = Array Size(array=w150) -> (size(s)=w167:i32)
            n238 = Decrement(x=w167) -> (x-1=w166:i32)
            n239 = Index Array(array=w150, index=w166) -> (element=w165:dbl)
            n240 = Index Array(array=w150, index=0) -> (element=w168:dbl)
            n241 = for {
              tunnel: w163 -> [w189]
              tunnel: w150 -> [_] mode=indexing
              tunnel: w158 -> [w185]
              tunnel: [w188] -> w170 mode=indexing
              tunnel: w168 -> [w187]
              tunnel: w150 -> [w186] mode=indexing
              n242 = call <vilib>:"Derivative x(t) PtByPt.vi"("initialize"=w189, "dt"=w185, "initial condition"=w187, "x"=w186) -> ("dx/dt"=w188:dbl)  [unwired: 1 out]
            }
            n243 = call <vilib>:"Derivative x(t) (obs).vi"("dt"=w158, "final condition"=w165, "initial condition"=w168, "X"=w150) -> ("dX/dt"=w160:dbl[])  [unwired: 1 out]
            n244 = Bundle("Value"=w159, w158, "Filtered X"=w150) -> (→"Smooth M.A.":cluster{"Value":dbl, dbl, "Filtered X":dbl[]})  [unwired: 1 in]
            n245 = Bundle("Value"=w159, w158, w170) -> ()  [unwired: 1 in, 1 out]
            n246 = Multiply(x=-2.302585093 ("y"), y=w160) -> (x*y=w151:dbl[])
            "y-axis" <- w151
            n247 = for {
              tunnel: w151 -> [w174] mode=indexing
              shift-right: [w175] -> w154
              shift-left: dbl[] [] ("Arrayin 2") -> [w176]
              n248 = Not A Number/Path/Refnum?(number/path/refnum=w174) -> (NaN/Path/Refnum?=w177:bool)
              n249 = case shown="True" w177 {
                tunnel: w176 -> [w180 w181]
                tunnel: [w179 w181] -> w175
                tunnel: w174 -> [w178 _]
                frame #0 {
                  n250 = Build Array (concatenate)(w180, w178) -> (w179:dbl[])
                }
                frame #1 {
                }
              }
            }
            n251 = Array Size(array=w154) -> (size(s)=w155:i32)
            n252 = for {
              tunnel: w158 -> [w184]
              shift-right: [w183] -> _
              shift-left: w159 -> [w182]
              tunnel: [w182] -> _ mode=indexing
              tunnel: w154 -> [_] mode=indexing
              n253 = Add(x=w184, y=w182) -> (x+y=w183:dbl)
            }
            n254 = Reshape Array(w154, w155) -> (w153:dbl[])
            n255 = Bundle("Filtered X"=w150, w151) -> (→"derivative M.A. 2":cluster{"Filtered X":dbl[], dbl[]})  [unwired: 1 in]
            n256 = Bundle("Value"=w159, w158, w151) -> (→"derivative M.A.":cluster{"Value":dbl, dbl, dbl[]})  [unwired: 1 in]
            n257 = call <vilib>:"Std Deviation and Variance.vi"("X"=w153) -> ("standard deviation"=→"S.D.":dbl)  [unwired: 1 in, 2 out]
          }
        }
        n258 = case shown="True" "Threshold?" {
          frame #0 {
          }
          frame #1 {
            w120 = T4 2 items=["Least Square", "Least Absolute Residual", "Bisquare"] ("method")
            n259 = property on="fit for M.A." class="WFGraph (strict)"() -> ("Value"=w130:cluster{"Value":dbl, dbl, dbl[]})  [unwired: 2 in, 2 out]
            n260 = Unbundle(w130) -> ("Value"=w118:dbl, w112:dbl, w110:dbl[])
            n261 = Negate(x=w110) -> (-x=w123:dbl[])
            n262 = Negate(x="threshold y 2") -> (-x=w121:dbl)
            n263 = Bundle("Value"=w118, w112, w110) -> (→"Threshold 2":cluster{"Value":dbl, dbl, dbl[]})  [unwired: 1 in]
            n264 = Threshold 1D Array(1:0 ("start index (0)"), 2:w121, 3:w123) -> (0:w127:dbl)
            n265 = Round Toward +Infinity(x=w127) -> (ceil(x): smallest int >= x=w126:dbl)
            n266 = Split 1D Array(array=w123, index=w126) -> (first subarray=w124:dbl[])  [unwired: 1 out]
            n267 = Negate(x=w124) -> (-x=w115:dbl[])
            n268 = Bundle("Value"=w118, w112, w115) -> (→"Real Threshold M.A.":cluster{"Value":dbl, dbl, dbl[]})  [unwired: 1 in]
            n269 = for {
              tunnel: [w131] -> w114 mode=indexing
              tunnel: w115 -> [_] mode=indexing
              i -> [w131]
            }
            n270 = To Double Precision Float(number=w114) -> (double precision float=w113:dbl[])
            n271 = Multiply(x=w112, y=w113) -> (x*y=w111:dbl[])
            n272 = call <vilib>:"Linear Fit.vi"("Y"=w115, "X"=w111, "method"=w120) -> ("Best Linear Fit"=w119:dbl[], "slope"=w108:dbl)  [unwired: 8 in, 3 out]
            n273 = Build Array(w115, w119) -> (w117:dbl[][])
            n274 = Bundle("Value"=w118, w112, w117) -> (→"fit for M.A 2":cluster{"Value":dbl, dbl, dbl[][]})  [unwired: 1 in]
            n275 = Multiply(x=w108, y=2.302585093) -> (x*y=→"slope M.A.":dbl)
          }
        }
      }
    }
  }
